vi "Log_comandos_aquisicion.vi"(8 "Estado":string, 9 "string de Resposta":string, 10 "string de comando":string, 11 "Porta":refnum<visa-resource-name>) -> ()   [LabVIEW 2012]
panel:
  out "Comando":string
  out "before substring":string
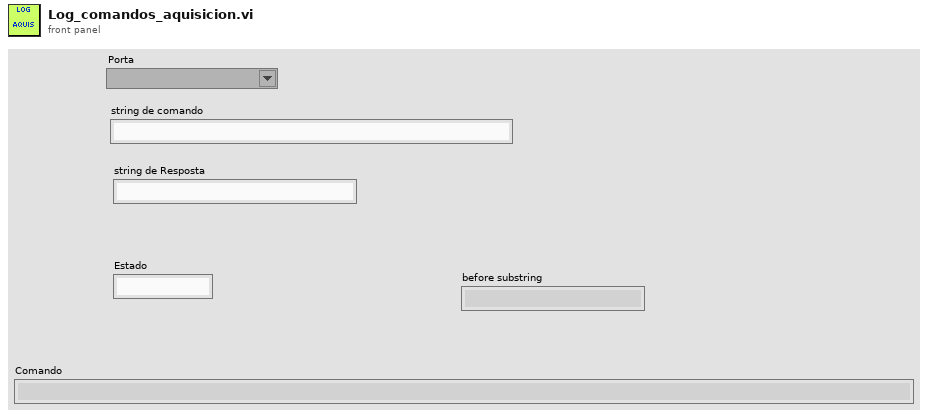
[diagram p1: front panel]
types:
  T1 = enum16{"open", "open or create", "create or replace", "create"}
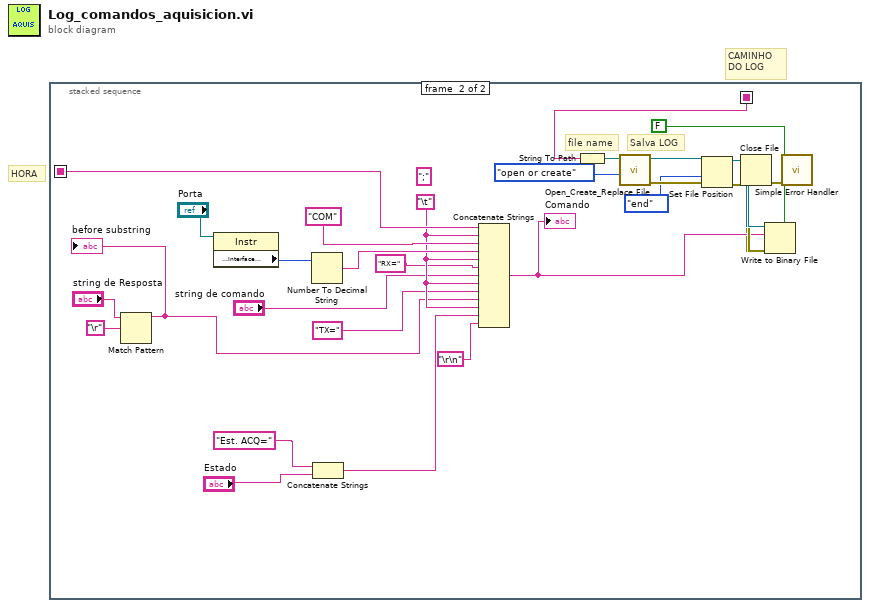
[diagram p0: block diagram]
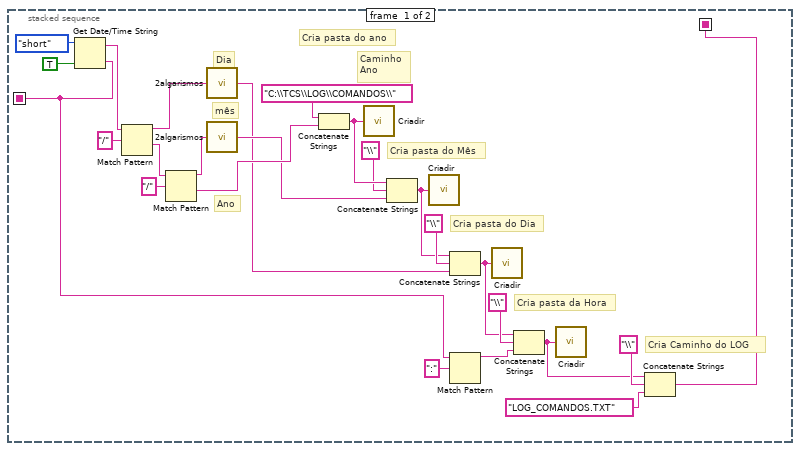
[diagram p2: hidden frame]
diagram:
  # "HORA"
  # "CAMINHO\nDO LOG"
  n1 = stacked-sequence {
    seq-local: [w9 _] -> [_ w40]
    seq-local: [w3 _] -> [_ w50]
    frame #0 {
      # "Cria pasta da Hora"
      # "Cria Caminho do LOG"
      # "Cria pasta do Dia"
      # "Cria pasta do Mês"
      # "Caminho\nAno"
      # "Ano"
      # "mês"
      # "Dia"
      # "Cria pasta do ano"
      n2 = Get Date/Time String(date format (0)=enum16{"short", "long", "abbreviated"}."short", want seconds? (F)=TRUE) -> (date string=w25:string, time string=w3:string)  [unwired: 1 in]
      n3 = Match Pattern(string=w25, regular expression="/") -> (before substring=w21:string, after substring=w22:string)  [unwired: 1 in, 2 out]
      n4 = Match Pattern(string=w22, regular expression="/") -> (before substring=w20:string, after substring=w18:string)  [unwired: 1 in, 2 out]
      n5 = call "2algarismos.vi"("entrada"=w21) -> ("saida"=w12:string)
      n6 = call "2algarismos.vi"("entrada"=w20) -> ("saida"=w15:string)
      n7 = Concatenate Strings("C:\\TCS\\LOG\\COMANDOS\\" ("SOMENTE DIRETORIO"), w18) -> (w17:string)
      n8 = call "Criadir.vi"("SOMENTE DIRETORIO"=w17) -> ()  [unwired: 2 out]
      n9 = Concatenate Strings(w17, "\\" ("regular expression"), w15) -> (w13:string)
      n10 = call "Criadir.vi"("SOMENTE DIRETORIO"=w13) -> ()  [unwired: 2 out]
      n11 = Concatenate Strings(w13, "\\" ("regular expression"), w12) -> (w5:string)
      n12 = Match Pattern(string=w3, regular expression=":") -> (before substring=w2:string)  [unwired: 1 in, 3 out]
      n13 = call "Criadir.vi"("SOMENTE DIRETORIO"=w5) -> ()  [unwired: 2 out]
      n14 = Concatenate Strings(w5, "\\" ("regular expression"), w2) -> (w1:string)
      n15 = call "Criadir.vi"("SOMENTE DIRETORIO"=w1) -> ()  [unwired: 2 out]
      n16 = Concatenate Strings(w1, "\\" ("regular expression"), "LOG_COMANDOS.TXT" ("regular expression")) -> (w9:string)
    }
    frame #1 {
      w36 = "\t"
      (unwired) ";"
      # "Salva LOG"
      # "file name"
      n17 = Match Pattern(string="string de Resposta", regular expression="\r") -> (before substring=w28:string)  [unwired: 1 in, 3 out]
      "before substring" <- w28
      n18 = property class="Instr"(reference="Porta") -> ("Interface Information:Interface Number"=w53:u16)  [unwired: 1 in, 2 out]
      n19 = Number To Decimal String(number=w53) -> (decimal integer string=w51:string)  [unwired: 1 in]
      n20 = Concatenate Strings("Est. ACQ=", "Estado") -> (w34:string)
      n21 = Concatenate Strings(w50, w36, "COM", w51, w36, "RX=", "string de comando", w36, "TX=", w28, w36, w34, "\r\n") -> (w41:string)
      "Comando" <- w41
      n22 = String To Path(string=w40) -> (path=w42:path)
      n23 = call <vilib>:"Open_Create_Replace File.vi"("function (open:0)"=T1."open or create", "file path"=w42) -> ("error out"=w45:errorcluster, "refnum"=w48:refnum<file>)  [unwired: 6 in, 2 out]
      n24 = Set File Position(refnum=w48, from (0:start)=enum16{"start", "end", "current"}."end" ("pos mode (0:2)"), error in=w45) -> (refnum out=w39:refnum<file>, error out=w38:errorcluster)  [unwired: 1 in]
      n25 = Write to Binary File(file (use dialog)=w39, data=w41, error in=w38, 5:FALSE ("prepend array or string size? (T)")) -> (refnum out=w47:refnum<file>, error out=w46:errorcluster)  [unwired: 2 in, 1 out]
      n26 = Close File(refnum=w47, error in=w46) -> (error out=w49:errorcluster)  [unwired: 1 out]
      n27 = call <vilib>:"Simple Error Handler.vi"("error in (no error)"=w49) -> ()  [unwired: 4 in, 5 out]
    }
  }
